vi "Frame Section Selection Screen.vi"(7 "guids":string[](array[string])=["4b95dee7-8d64-48ce-932c-f5fdd14e4d4c", "94e87467-031b-484c-a85e-bcbac581524d"], 8 "error in":errorcluster, 11 "Parent Ref":T2=18446744073709551615 format="%.0x") -> (0 "error out":errorcluster, 1 "Cancelled?":bool, 2 "Output Selections":T1[](array[typedef]) {"Node Ref" format="%.0x"}, 3 "Parent Ref Out":T2=18446744073709551615 format="%.0x")   [LabVIEW 2023, in "Protection and Counter Support System Explorer.lvlib"]
uses:
  Protection and Counter Support System Explorer.lvlib
  <vilib>/NI VeriStand/Custom Device API/Custom Device API.lvlib
  <vilib>/NI VeriStand/Custom Device API/Custom Device Item Ref.ctl
  Types/Protection Signal Linked Channel.ctl
  NationalInstruments.VeriStand.SystemStorageUI
panel:
  in  "Cancel":bool
  in  "OK":bool
  in  "Protection Data":refnum<k24>(container)
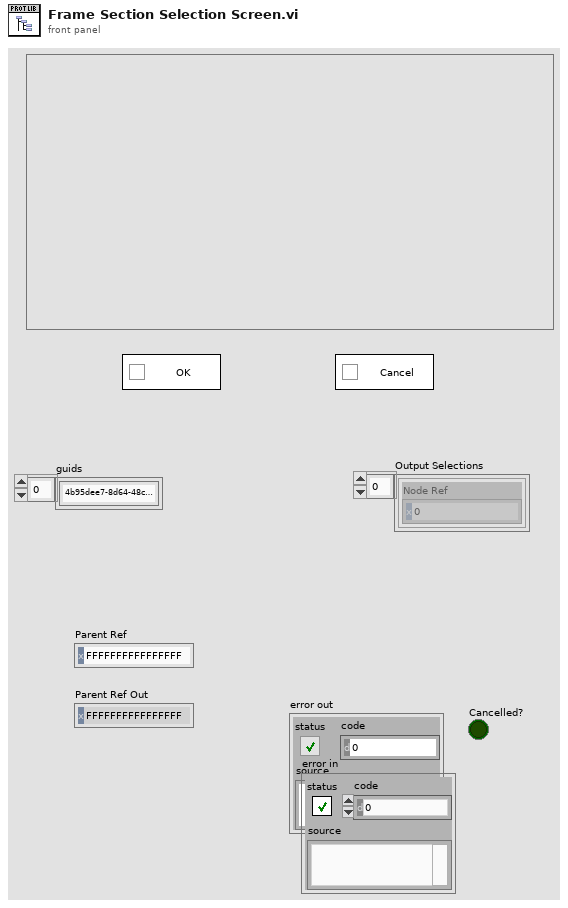
[diagram p1: front panel]
types:
  T1 = typedef "Protection and Counter Support System Explorer.lvlib/Protection Signal Linked Channel.ctl" = cluster{"Node Ref":T2}
  T2 = typedef "Custom Device API.lvlib/Custom Device Item Ref.ctl" = u64
  T3 = typedef "Custom Device API.lvlib/Custom Device Pointer.ctl" = refnum<k24>
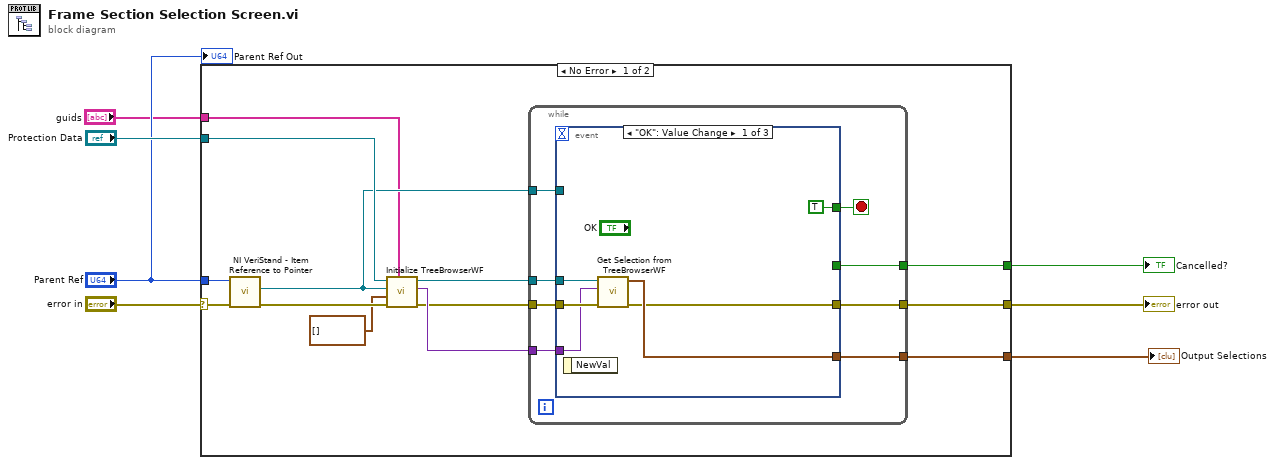
[diagram p0: block diagram]
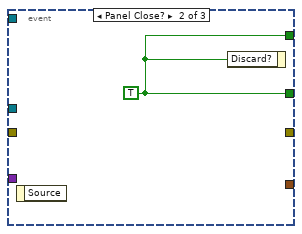
[diagram p2: hidden frame]
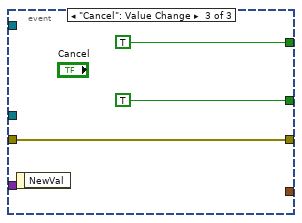
[diagram p3: hidden frame]
diagram:
  n1 = case shown="No Error" "error in" {
    selector: "error in" -> [w19 w39]
    tunnel: "Protection Data" -> [w16 _]
    tunnel: "Parent Ref" -> [w20 _]
    tunnel: [w18 _] -> w6
    tunnel: [w13 w39] -> w5
    tunnel: [w17 _] -> w1
    tunnel: "guids" -> [w9 _]
    frame No Error {
      n2 = call <vilib>:"NI VeriStand - Item Reference to Pointer.vi"("error in (no error)"=w19, "Item Ref in"=w20) -> ("error out"=w12:errorcluster, "Node Pointer"=w11:T3)  [unwired: 6 in, 2 out]
      n3 = call "Initialize TreeBrowserWF.vi"("guids"=w9, "error in (no error)"=w12, "Input Channels"=cluster{"Node ID":u64}[] [], "Node Pointer"=w11, "TreeBrowserRef"=w16) -> ("error out"=w10:errorcluster, "Channels"=w15:variant, "TreeBrowserRef 2"=w14:refnum<k24>)  [unwired: 4 in]
      n4 = while {
        tunnel: w10 -> [w28]
        tunnel: w14 -> [w27]
        tunnel: [w25] -> w18
        tunnel: [w24] -> w13
        tunnel: [w23] -> w17
        tunnel: w15 -> [w22]
        tunnel: w11 -> [w21]
        stop <- w26 stop-if-true
        n5 = event shown="[0] \"OK\": Value Change" {
          selector: _ -> [_ _ _]
          dyn-events: _ -> [_ _ _]
          timeout: _ -> [_ _ _]
          tunnel: w28 -> [w34 _ w38]
          tunnel: w27 -> [w33 _ _]
          tunnel: [w30 _ w38] -> w24
          tunnel: [TRUE w35 TRUE] -> w26
          tunnel: [_ w35 TRUE] -> w25
          tunnel: [w31 _ _] -> w23
          tunnel: w22 -> [w32 _ _]
          tunnel: w21 -> [_ _ _]
          event "OK": Value Change {
            n6 = event-data() -> ()  [unwired: 1 in, 1 out]
            n7 = call "Get Selection from TreeBrowserWF.vi"("error in (no error)"=w34, "Input Channels"=w32, ".NET Refnum in"=w33) -> ("error out"=w30:errorcluster, "Input Channel Selections"=w31:T1[])  [unwired: 7 in]
          }
          event Panel Close? {
            w35 = TRUE
            n8 = event-data() -> ()  [unwired: 1 in, 1 out]
            n9 = event-data("Discard?"=w35) -> ()  [unwired: 1 in, 1 out]
          }
          event "Cancel": Value Change {
            n10 = event-data() -> ()  [unwired: 1 in, 1 out]
          }
        }
      }
    }
    frame Error {
    }
  }
  "Cancelled?" <- w6
  "error out" <- w5
  "Output Selections" <- w1
  "Parent Ref Out" <- "Parent Ref"
